vi "steering_velocity_generation.vi"(8 "angular velocity":dbl, 9 "forward velocity":dbl, 11 "bool-to-dec value":dbl) -> (0 "motor_control_sig":string, 2 "angular velocity 2":i32, 3 "forward velocity 2":i32)   [LabVIEW 2012]
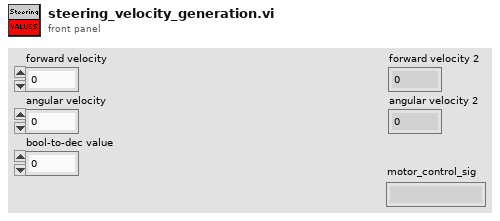
[diagram p1: front panel]
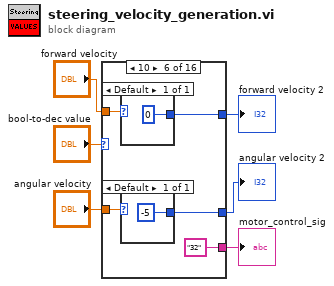
[diagram p0: block diagram]
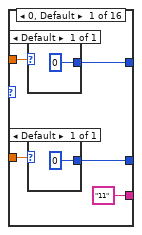
[diagram p2: hidden frame]
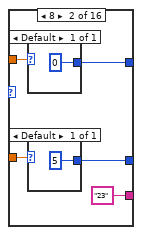
[diagram p3: hidden frame]
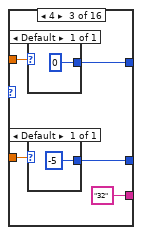
[diagram p4: hidden frame]
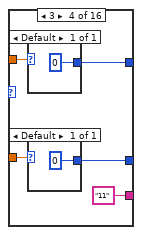
[diagram p5: hidden frame]
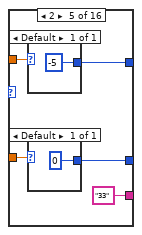
[diagram p6: hidden frame]
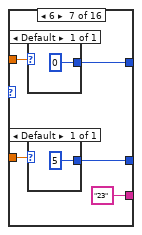
[diagram p7: hidden frame]
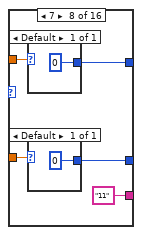
[diagram p8: hidden frame]
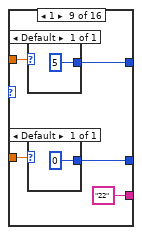
[diagram p9: hidden frame]
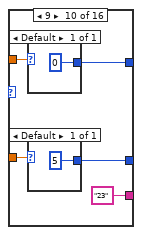
[diagram p10: hidden frame]
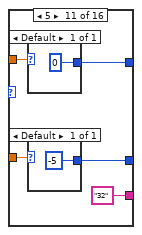
[diagram p11: hidden frame]
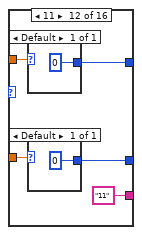
[diagram p12: hidden frame]
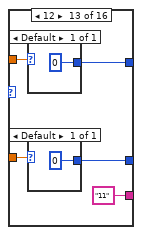
[diagram p13: hidden frame]
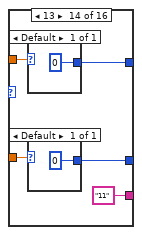
[diagram p14: hidden frame]
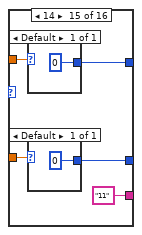
[diagram p15: hidden frame]
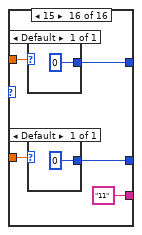
[diagram p16: hidden frame]
diagram:
  n1 = case shown="10" "bool-to-dec value" {
    tunnel: [w8 w15 w22 w31 w39 w43 w50 w57 w65 w72 w78 w87 w93 w99 w107 w113] -> w2
    tunnel: "forward velocity" -> [w11 w18 w25 w32 w36 w46 w53 w60 w66 w74 w81 w86 w94 w102 w108 w116]
    tunnel: "angular velocity" -> [w10 w17 w24 w29 w37 w45 w52 w59 w67 w73 w80 w85 w95 w101 w109 w115]
    tunnel: [w9 w16 w23 w30 w38 w44 w51 w58 w64 w71 w79 w88 w92 w100 w106 w114] -> w4
    tunnel: ["11" ("motor_control_sig") "23" ("motor_control_sig") "32" ("motor_control_sig") "11" ("motor_control_sig") "33" ("motor_control_sig") "32" ("motor_control_sig") "23" ("motor_control_sig") "11" ("motor_control_sig") "22" ("motor_control_sig") "23" ("motor_control_sig") "32" ("motor_control_sig") "11" ("motor_control_sig") "11" ("motor_control_sig") "11" ("motor_control_sig") "11" ("motor_control_sig") "11" ("motor_control_sig")] -> w1
    frame 0, Default {
      n2 = case shown="Default" w11 {
        tunnel: [0] -> w8
        frame Default {
        }
      }
      n3 = case shown="Default" w10 {
        tunnel: [0] -> w9
        frame Default {
        }
      }
    }
    frame 8 {
      n4 = case shown="Default" w18 {
        tunnel: [0] -> w15
        frame Default {
        }
      }
      n5 = case shown="Default" w17 {
        tunnel: [5] -> w16
        frame Default {
        }
      }
    }
    frame 4 {
      n6 = case shown="Default" w25 {
        tunnel: [0] -> w22
        frame Default {
        }
      }
      n7 = case shown="Default" w24 {
        tunnel: [-5] -> w23
        frame Default {
        }
      }
    }
    frame 3 {
      n8 = case shown="Default" w32 {
        tunnel: [0] -> w31
        frame Default {
        }
      }
      n9 = case shown="Default" w29 {
        tunnel: [0] -> w30
        frame Default {
        }
      }
    }
    frame 2 {
      n10 = case shown="Default" w36 {
        tunnel: [-5] -> w39
        frame Default {
        }
      }
      n11 = case shown="Default" w37 {
        tunnel: [0] -> w38
        frame Default {
        }
      }
    }
    frame 10 {
      n12 = case shown="Default" w46 {
        tunnel: [0] -> w43
        frame Default {
        }
      }
      n13 = case shown="Default" w45 {
        tunnel: [-5] -> w44
        frame Default {
        }
      }
    }
    frame 6 {
      n14 = case shown="Default" w53 {
        tunnel: [0] -> w50
        frame Default {
        }
      }
      n15 = case shown="Default" w52 {
        tunnel: [5] -> w51
        frame Default {
        }
      }
    }
    frame 7 {
      n16 = case shown="Default" w60 {
        tunnel: [0] -> w57
        frame Default {
        }
      }
      n17 = case shown="Default" w59 {
        tunnel: [0] -> w58
        frame Default {
        }
      }
    }
    frame 1 {
      n18 = case shown="Default" w66 {
        tunnel: [5] -> w65
        frame Default {
        }
      }
      n19 = case shown="Default" w67 {
        tunnel: [0] -> w64
        frame Default {
        }
      }
    }
    frame 9 {
      n20 = case shown="Default" w74 {
        tunnel: [0] -> w72
        frame Default {
        }
      }
      n21 = case shown="Default" w73 {
        tunnel: [5] -> w71
        frame Default {
        }
      }
    }
    frame 5 {
      n22 = case shown="Default" w81 {
        tunnel: [0] -> w78
        frame Default {
        }
      }
      n23 = case shown="Default" w80 {
        tunnel: [-5] -> w79
        frame Default {
        }
      }
    }
    frame 11 {
      n24 = case shown="Default" w86 {
        tunnel: [0] -> w87
        frame Default {
        }
      }
      n25 = case shown="Default" w85 {
        tunnel: [0] -> w88
        frame Default {
        }
      }
    }
    frame 12 {
      n26 = case shown="Default" w94 {
        tunnel: [0] -> w93
        frame Default {
        }
      }
      n27 = case shown="Default" w95 {
        tunnel: [0] -> w92
        frame Default {
        }
      }
    }
    frame 13 {
      n28 = case shown="Default" w102 {
        tunnel: [0] -> w99
        frame Default {
        }
      }
      n29 = case shown="Default" w101 {
        tunnel: [0] -> w100
        frame Default {
        }
      }
    }
    frame 14 {
      n30 = case shown="Default" w108 {
        tunnel: [0] -> w107
        frame Default {
        }
      }
      n31 = case shown="Default" w109 {
        tunnel: [0] -> w106
        frame Default {
        }
      }
    }
    frame 15 {
      n32 = case shown="Default" w116 {
        tunnel: [0] -> w113
        frame Default {
        }
      }
      n33 = case shown="Default" w115 {
        tunnel: [0] -> w114
        frame Default {
        }
      }
    }
  }
  "forward velocity 2" <- w2
  "angular velocity 2" <- w4
  "motor_control_sig" <- w1
